vi "test_libssh2_session_methods.vi"() -> ()   [LabVIEW 2013, in "libssh2_integration_tests.lvlib"]
uses:
  libssh2_integration_tests.lvlib
  libssh2/libssh2_method_type.ctl
  <vilib>/addons/_JKI Toolkits/Caraya/classes/Test/Test.lvclass
  libssh2/libssh2.lvlib
  <vilib>/addons/_JKI Toolkits/Caraya/classes/Assert/Assert.lvclass
panel:
  out "error out":errorcluster
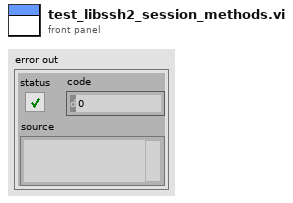
[diagram p1: front panel]
types:
  T1 = typedef "libssh2.lvlib/libssh2_method_type.ctl" = enum16{"LIBSSH2_METHOD_KEX", "LIBSSH2_METHOD_HOSTKEY", "LIBSSH2_METHOD_CRYPT_CS", "LIBSSH2_METHOD_CRYPT_SC", "LIBSSH2_METHOD_MAC_CS", "LIBSSH2_METHOD_MAC_SC", "LIBSSH2_METHOD_COMP_CS", "LIBSSH2_METHOD_COMP_SC", "LIBSSH2_METHOD_LANG_CS", "LIBSSH2_METHOD_LANG_SC", "LIBSSH2_METHOD_SIGN_ALGO"}
  T2 = typedef "libssh2.lvlib/Session Refnum.ctl" = refnum<k1>
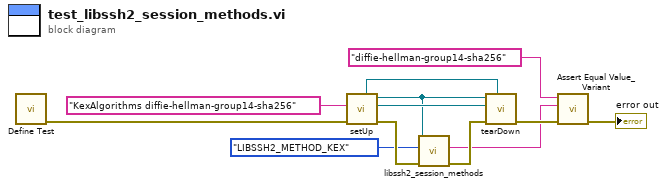
[diagram p0: block diagram]
diagram:
  n1 = call <vilib>:"Define Test.vi"() -> ("error out"=w12:errorcluster)  [unwired: 10 in, 1 out]
  n2 = call "setUp.vi"("error in (no error)"=w12, "sshd_config"="KexAlgorithms diffie-hellman-group14-sha256") -> ("error out"=w6:errorcluster, "connection ID"=w10:refnum<k5>, "session"=w8:T2, "fixture"=w9:refnum<class "Server Fixture.lvclass">)  [unwired: 6 in]
  n3 = call "libssh2_session_methods.vi"("error in (no error)"=w6, "method_type"=libssh2_method_type."LIBSSH2_METHOD_KEX", "session"=w8) -> ("error out"=w7:errorcluster, "methods"=w4:string)  [unwired: 7 in]
  n4 = call "tearDown.vi"("fixture"=w9, "error in (no error)"=w7, "connection ID"=w10, "session"=w8) -> ("error out"=w5:errorcluster)  [unwired: 7 in]
  n5 = call <vilib>:"Assert Equal Value_Variant.vi"("error in (no error)"=w5, "Y"=w4, "X"="diffie-hellman-group14-sha256") -> ("error out"=→"error out":errorcluster)  [unwired: 7 in, 1 out]
